vi "zmq_request_socket.vi"() -> ()   [LabVIEW 2014]
uses:
  <vilib>/addons/zeromq/socket_type.ctl
  <vilib>/addons/zeromq/zmq_context.lvclass
  <vilib>/addons/zeromq/zmq_socket.lvclass
  <vilib>/addons/zeromq/zeromq.lvlib
panel:
  in  "dimension size 2":i32=1
  in  "dimension size":i32=4
  out "value":dbl[][](array[numeric])
  out "Array sent from LV":dbl[][](array[numeric])
  in  "Array value":dbl=1234.56 format="%#_13g"
  in  "Send Array (on)\nSend String (off)":bool
  in  "Message":string="hello"
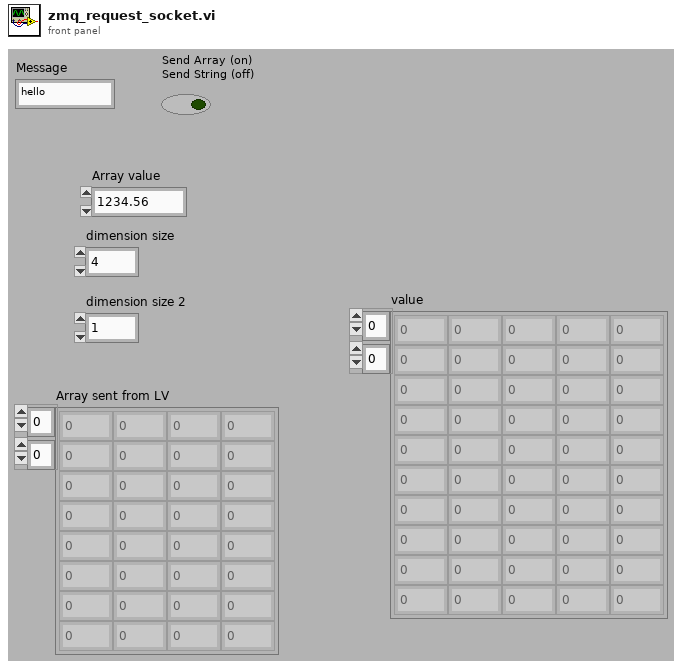
[diagram p1: front panel]
types:
  T1 = enum16{"big-endian, network order", "native, host order", "little-endian"}
  T2 = typedef "zeromq.lvlib/socket_type.ctl" = enum8{"ZMQ_PAIR", "ZMQ_PUB", "ZMQ_SUB", "ZMQ_REQ", "ZMQ_REP", "ZMQ_DEALER", "ZMQ_ROUTER", "ZMQ_PULL", "ZMQ_PUSH", "ZMQ_XPUB", "ZMQ_XSUB"}
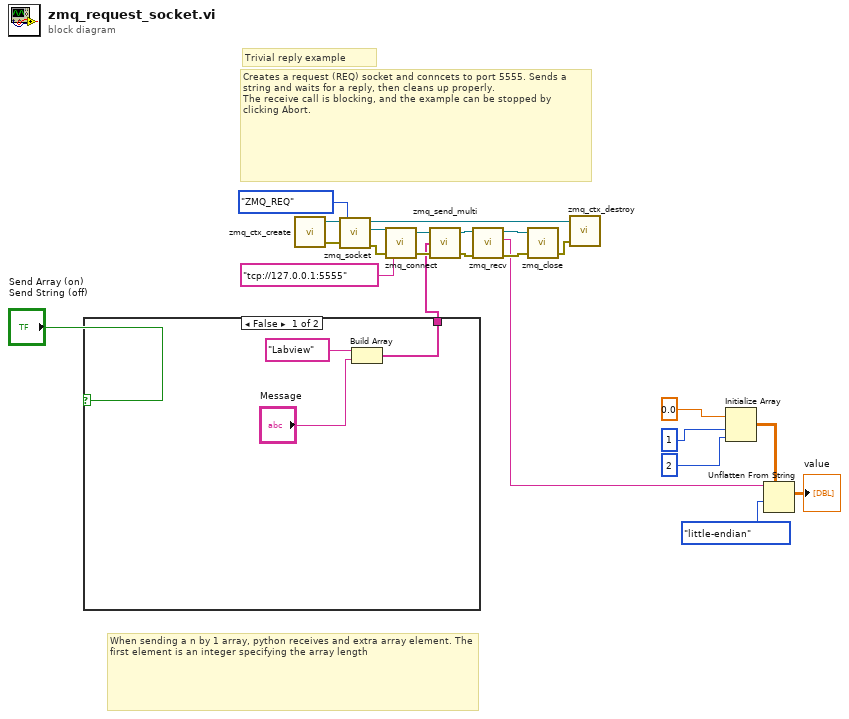
[diagram p0: block diagram]
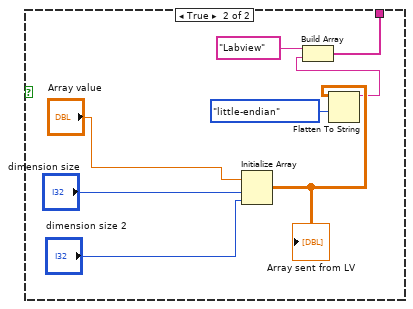
[diagram p2: hidden frame]
diagram:
  # "When sending a n by 1 array, python receives and extra array element. The first element is an integer specifying the array length"
  # "Creates a request (REQ) socket and conncets to port 5555. Sends a string and waits for a reply, then cleans up properly.\nThe receive call is blocking, and the example can be stopped by clicking Abort."
  # "Trivial reply example"
  n1 = case shown="False" "Send Array (on)\nSend String (off)" {
    tunnel: [w24 w27] -> w5
    frame False {
      n2 = Build Array("Labview", "Message") -> (w24:string[])
    }
    frame True {
      n3 = Initialize Array("Array value", "dimension size", "dimension size 2") -> (w31:dbl[][])
      "Array sent from LV" <- w31
      n4 = Flatten To String(anything=w31, byte order (0:big-endian, network order)=T1."little-endian") -> (data string=w28:string)  [unwired: 2 in, 2 out]
      n5 = Build Array("Labview", w28) -> (w27:string[])
    }
  }
  n6 = call <vilib>:"zmq_ctx_create.vi"() -> ("error out"=w13:errorcluster, "context out"=w23:refnum<class "zmq_context.lvclass">)  [unwired: 4 in]
  n7 = call <vilib>:"zmq_socket.vi"("error in"=w13, "socket type"=socket_type."ZMQ_REQ", "context in"=w23) -> ("error out"=w22:errorcluster, "socket out"=w21:refnum<class "zmq_socket.lvclass">, "context out"=w14:refnum<class "zmq_context.lvclass">)  [unwired: 2 in]
  n8 = call <vilib>:"zmq_connect.vi"("error in"=w22, "endpoint"="tcp://127.0.0.1:5555", "socket in"=w21) -> ("error out"=w20:errorcluster, "socket out"=w19:refnum<class "zmq_socket.lvclass">)  [unwired: 1 in]
  n9 = call <vilib>:"zmq_send_multi.vi"("error in"=w20, "parts"=w5, "socket in"=w19) -> ("error out"=w12:errorcluster, "socket out"=w18:refnum<class "zmq_socket.lvclass">)  [unwired: 1 in]
  n10 = call <vilib>:"zmq_recv.vi"("error in"=w12, "socket in"=w18) -> ("error out"=w17:errorcluster, "data"=w1:string, "socket out"=w16:refnum<class "zmq_socket.lvclass">)  [unwired: 3 in, 2 out]
  n11 = call <vilib>:"zmq_close.vi"("error in"=w17, "socket"=w16) -> ("error out"=w15:errorcluster)  [unwired: 3 in]
  n12 = call <vilib>:"zmq_ctx_destroy.vi"("error in"=w15, "context in"=w14) -> ()  [unwired: 3 in, 1 out]
  n13 = Initialize Array(0.0, 1 ("dimension size"), 2 ("dimension size")) -> (w3:dbl[][])
  n14 = Unflatten From String(type=w3, binary string=w1, byte order (0:big-endian, network order)=T1."little-endian") -> (value=→"value":dbl[][])  [unwired: 2 in, 2 out]
